vi "Start.vi"(7 "Buffer Size (4096)":i32=4096, 8 "error in (no error)":errorcluster, 11 "Mixer in":refnum<class "Mixer.lvclass">) -> (0 "error out":errorcluster, 3 "Mixer out":refnum<class "Mixer.lvclass">)   [LabVIEW 2020, in "G-Audio.lvlib" / "Mixer.lvclass"]
uses:
  Mixer.lvclass
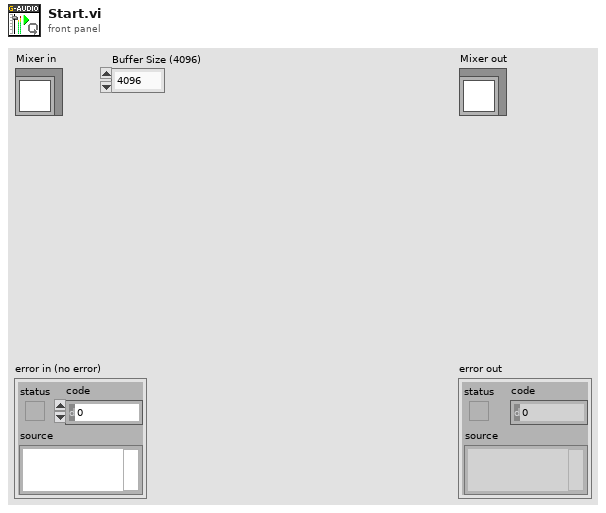
[diagram p1: front panel]
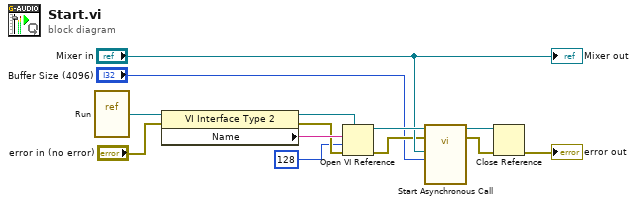
[diagram p0: block diagram]
diagram:
  n1 = vi-ref "Run.vi"() -> (w13:refnum<vi>)
  n2 = property class="VI Interface Type 2"(reference=w13, error in="error in (no error)") -> (reference out=w11:refnum<vi>, error out=w7:errorcluster, "Name"=w12:string)
  n3 = Open VI Reference(type specifier VI Refnum (for type only)=w11, vi path=w12, options=128, error in (no error)=w7) -> (vi reference=w10:refnum<vi>, error out=w6:errorcluster)  [unwired: 2 in]
  n4 = call-by-ref "Start Asynchronous Call"(reference=w10, error in=w6, "Buffer Size"="Buffer Size (4096)", "Mixer in"="Mixer in") -> (reference out=w2:refnum<vi>, error out=w5:errorcluster)  [unwired: 9 in, 1 out]
  n5 = Close Reference(reference=w2, error in (no error)=w5) -> (error out=→"error out":errorcluster)
  "Mixer out" <- "Mixer in"
